vi "Config Counter to Measure Two Edge Separation.vi"(8 "errIN":errorcluster, 9 "SampClk.Timebase.Src":tag="/LightScreens/80MHzTimebase", 11 "Counter":tag="Dev1/ctr0") -> (0 "errOUT":errorcluster, 3 "task out":refnum<k21>)   [LabVIEW 2015]
doc: "DESCRIPTION:\nThis VI arms two counters, using an NI-TIO based device (e.g.: 6602). The counters increments its event count everytime a pulse comes into its source input. The counters only increments between the rising edge of the aux line and the rising edge of the gate. The value of the counter can be read when the counter is finished or an error occurs. \n\n\n\nINSTRUCTIONS:\n1. Enter the device and counter you want use.\n\n3. Connect your signals as described below in I/O CONNECTIONS.\n4. Run the VI.\n\n\nKEY PARAMETERS:\nCounter Group Config.vi: task type = two edge separation measurement\nCounter Source (NI-TIO).vi: Source Specification\nCounter Gate (NI-TIO).vi: Gate Specification\nCounter Aux Line (NI-TIO): Aux Line Specification\nCounter Get Attribute.vi: armed, TC Reached, count\nCounter Control.vi: Program, Reset\n\n\n\nI/O CONNECTIONS:\nConnect the start signal to the aux line input of the selected counter. Connect the stop signal to the gate input of the selected counter. \nIf you selected the Source Selection to be \"PFI line\", connect your event count base signal to the PFI line indicated by \"Source PFI line number used\". (If you selected \"Internal Timebase\", no source connection is necessary.)\n\nNOTE: For actual I/O pin numbers, please refer to your hardware user manual.\n\n\n\nDAQ VIs USED:\nCounter Group Config.vi\nCounter Source (NI-TIO).vi\nCounter Gate (NI-TIO).vi\nCounter Aux Line (NI-TIO)\nCounter Get Attribute.vi\nCounter Control.vi"
uses:
  <vilib>/DAQmx/create/channels.llb/DAQmx Create Channel (CI-Two Edge Separation).vi
  <resource>/objmgr/daqmx.rc
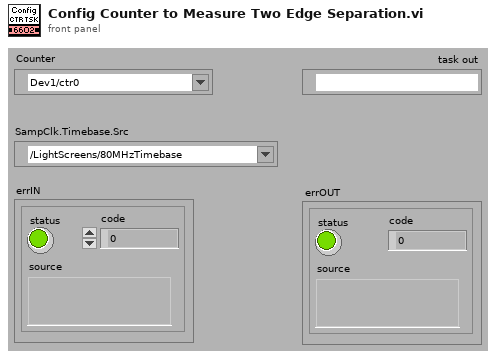
[diagram p1: front panel]
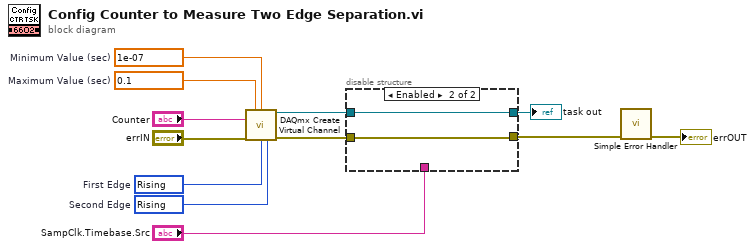
[diagram p0: block diagram]
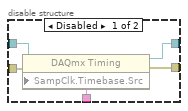
[diagram p2: hidden frame]
diagram:
  w8 = 10280 items=["Rising"=10280, "Falling"=10171]  # Second Edge
  w9 = 10280 items=["Rising"=10280, "Falling"=10171]  # First Edge
  w11 = 0.1  # Maximum Value (sec)
  w10 = 1e-07  # Minimum Value (sec)
  n1 = call-poly <vilib>:"DAQmx Create Virtual Channel.vi"("maximum value"=w11, "minimum value"=w10, "counter"="Counter", "error in"="errIN", "first edge"=w9, "second edge"=w8) -> ("task out"=w4:refnum<k21>, "error out"=w5:errorcluster)  [unwired: 8 in]
  n2 = disable-structure shown="Enabled" {
    disable-tunnel: "SampClk.Timebase.Src" -> [w17 _]
    disable-tunnel: w5 -> [w16 w18]
    disable-tunnel: w4 -> [w15 w19]
    disable-tunnel: [w14 w18] -> w3
    disable-tunnel: [w13 w19] -> w2
    frame Disabled {
      n3 = property class="DAQmx Timing"(reference=w15, error in=w16, "SampClk.Timebase.Src"=w17) -> (reference out=w13:refnum<k21>, error out=w14:errorcluster)
    }
    frame Enabled {
    }
  }
  "task out" <- w2
  n4 = call <vilib>:"Simple Error Handler.vi"("error in (no error)"=w3) -> ("error out"=→"errOUT":errorcluster)  [unwired: 4 in, 4 out]
